vi "Init Actor Core.vi"(8 "error in (no error)":errorcluster, 11 "Mag Lab Measure Interface in":refnum<class "XY Plot.lvclass">) -> (0 "error out":errorcluster, 3 "Mag Lab Measure Interface out":refnum<class "XY Plot.lvclass">)   [LabVIEW 2019, in "XY Plot.lvclass"]
uses:
  XY Plot.lvclass
  Plot/Plot.lvclass
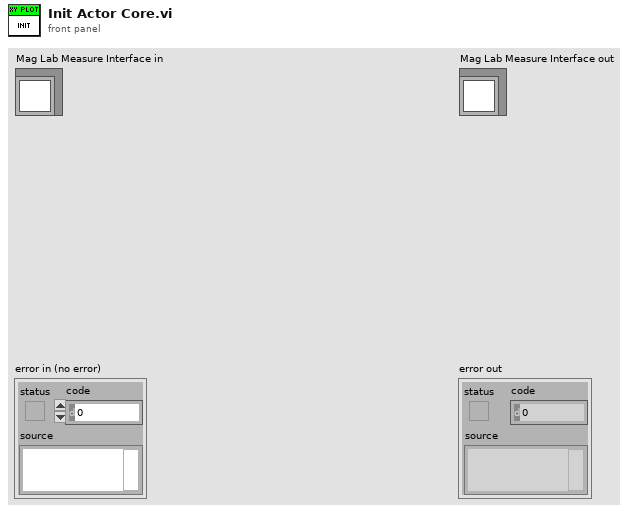
[diagram p1: front panel]
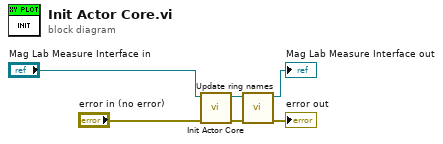
[diagram p0: block diagram]
diagram:
  n1 = call-parent "Init Actor Core.vi"("error in (no error)"="error in (no error)", "Measure Object in"="Mag Lab Measure Interface in") -> ("error out"=w1:errorcluster, "Measure Object out"=w3:refnum<class "XY Plot.lvclass">)  [unwired: 8 in]
  n2 = call "Update ring names.vi"("error in (no error)"=w1, "MagLabGraph in"=w3) -> ("error out"=→"error out":errorcluster, "MagLabGraph out"=→"Mag Lab Measure Interface out":refnum<class "XY Plot.lvclass">)  [unwired: 8 in]
